vi "ConcatTwoArrayOfStrings.vi"(9 "Array 2":string[](array[string]), 11 "Array":string[](array[string])) -> (3 "Array 3":string[](array[string]))   [LabVIEW 2012]
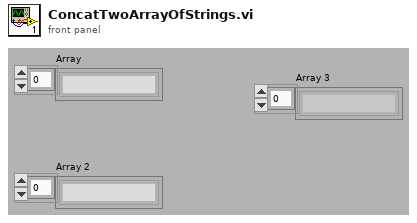
[diagram p1: front panel]
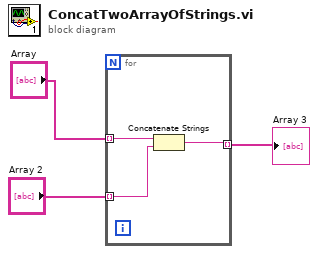
[diagram p0: block diagram]
diagram:
  n1 = for {
    tunnel: [w6] -> w3 mode=indexing
    tunnel: "Array" -> [w5] mode=indexing
    tunnel: "Array 2" -> [w4] mode=indexing
    n2 = Concatenate Strings(w5, w4) -> (w6:string)
  }
  "Array 3" <- w3
